vi "TechnosoftVariables.vi"(0 "error in (no error)":errorcluster) -> (1 "error out":errorcluster, 3 "Decoded new":bool, 4 "TSM variable table":T1 {"?" format="%x"})   [LabVIEW 8.6]
panel:
  out "Number of variables":i32
  out "Numeric":i32
  out "decode":string
  out "Unknown type String":string
  in  "Firmware variables.cfg":string
  # "Store as a constant!\nMap data 0000-FFFF\nEPROM: 10000-1FFFF\nTSM prog: 20000-2FFFF"
  # "TSM Data: 200-3FF and 800-9FF-FFF, 8000-FFFF(external)\nTSM prog: 8000-FFFF\nEPROM:  4000-7FFF"
  # "In the Technosoft manual all real variables are CAPITAL letters,\nso do it here."
  # "checked with old dataset: i2tintlim_m and other _m"
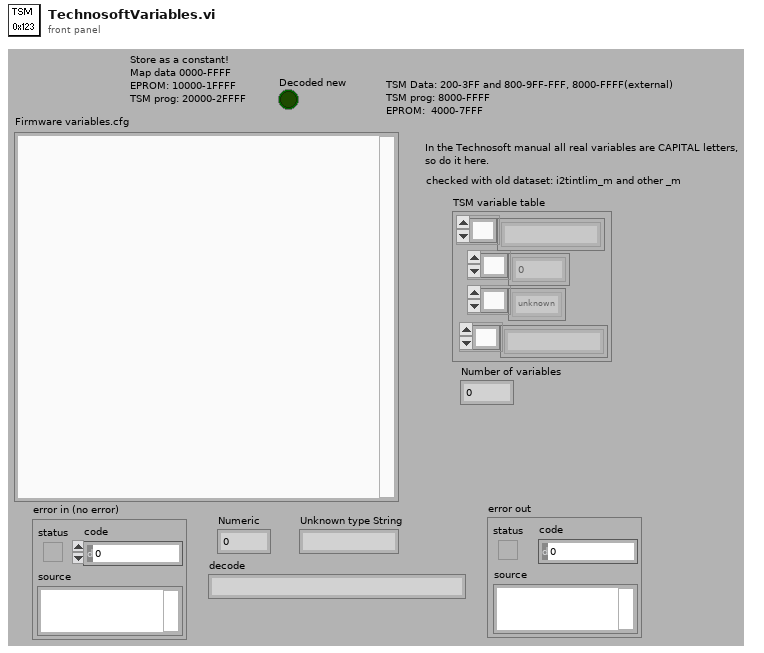
[diagram p1: front panel]
types:
  T1 = cluster{string[], u32[], enum16{"unknown", "i16", "u16", "i32", "u32", "fix32"}[], "comment":string[]}
  T2 = cluster{"String 1":string, i32, "type":enum16{"unknown", "i16", "u16", "i32", "u32", "fix32"}, "trimmed string":string}[]
  T3 = enum16{"unknown", "i16", "u16", "i32", "u32", "fix32"}[]
  T4 = enum16{"unknown", "i16", "u16", "i32", "u32", "fix32"}
  T5 = cluster{string, "Address":u32, "type":enum16{"unknown", "i16", "u16", "i32", "u32", "fix32"}, "trimmed string":string}
  T6 = cluster{"String 1":string, "Address":u32, "type":enum16{"unknown", "i16", "u16", "i32", "u32", "fix32"}, "trimmed string":string}[]
  T7 = cluster{string[], u32[], enum16{"unknown", "i16", "u16", "i32", "u32", "fix32"}[], string[]}
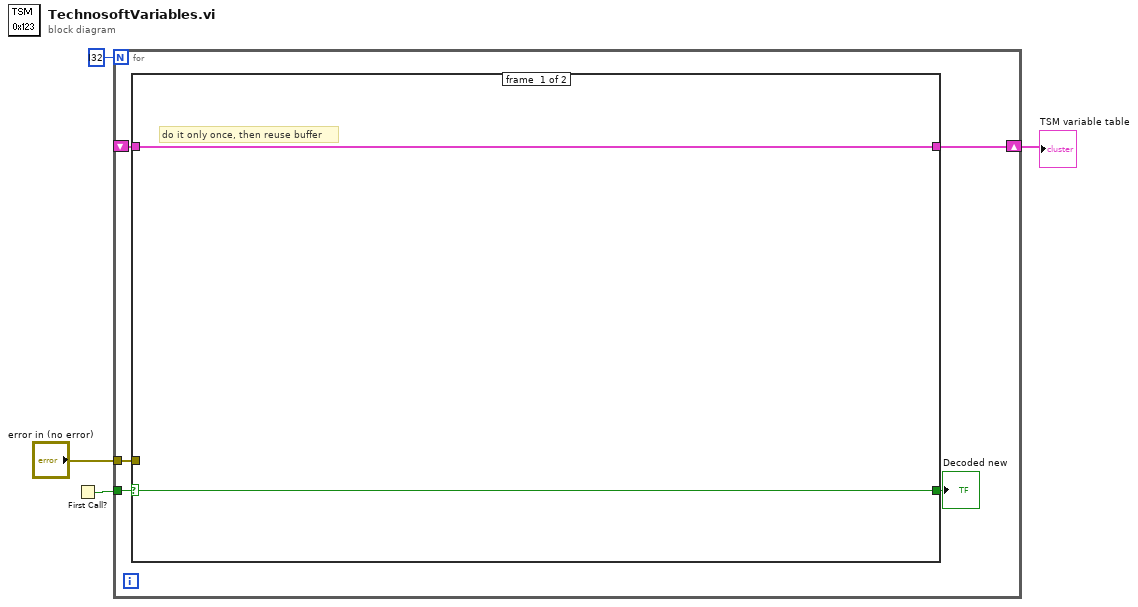
[diagram p0: block diagram]
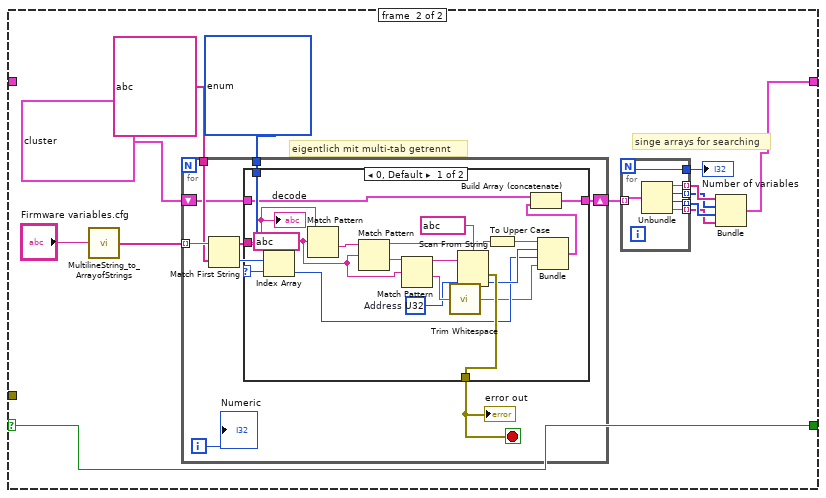
[diagram p2: hidden frame]
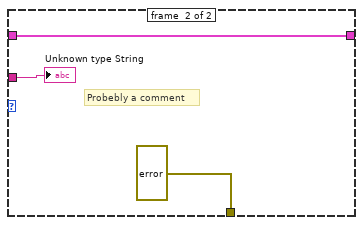
[diagram p3: hidden frame]
diagram:
  n1 = First Call?() -> (First Call?: T/F=w4:bool)
  n2 = for {
    N: i32 ? -> [_]
    tunnel: w4 -> [w9]
    tunnel: "error in (no error)" -> [w7]
    shift-right: [w6] -> w2
    shift-left: _ -> [w5]
    n3 = case shown="True" w9 {
      selector: w9 -> [w11 w20]
      tunnel: [w11 w20] -> w8
      tunnel: w7 -> [_ _]
      tunnel: [w10 w13] -> w6
      tunnel: w5 -> [w10 _]
      frame #0 {
        # "do it only once, then reuse buffer"
      }
      frame #1 {
        w21 = T3 ? items=["unknown", "i16", "u16", "i32", "u32", "fix32"]
        # "singe arrays for searching"
        # "eigentlich mit multi-tab getrennt"
        n4 = call "MultilineString_to_ArrayofStrings.vi"("String 1"="Firmware variables.cfg") -> ("String Array"=w23:string[])  [unwired: 1 in]
        n5 = for {
          tunnel: w23 -> [w39] mode=indexing
          tunnel: string[] ? -> [w38]
          tunnel: w21 -> [w35]
          shift-right: [w32] -> w18
          shift-left: T2 ? -> [w31]
          i -> [w33]
          stop <- w34 stop-if-true
          n6 = Match First String(2:w38, 3:w39) -> (0:w37:i32, 1:w36:string)
          n7 = case shown="0, Default" w37 {
            selector: w37 -> [w57 _]
            tunnel: w36 -> [w56 w61]
            tunnel: w35 -> [w58 _]
            tunnel: [w49 errorcluster ? ("error IO")] -> w34
            tunnel: [w46 w59] -> w32
            tunnel: w31 -> [w43 w59]
            frame #0 {
              w42 = u32 ?  # Address
              w53 = string ? ("regular expression")
              n8 = Index Array(array=w58, index=w57) -> (element=w45:T4)
              n9 = Match Pattern(string=w56, regular expression=w53) -> (after substring=w55:string)  [unwired: 4 out]
              n10 = Match Pattern(string=w55, regular expression=w53) -> (before substring=w41:string, after substring=w54:string)  [unwired: 3 out]
              n11 = Match Pattern(string=w54, regular expression=w53) -> (before substring=w51:string, after substring=w52:string)  [unwired: 3 out]
              n12 = call <vilib>:"Trim Whitespace.vi"("string"=w52) -> ("trimmed string"=w44:string)  [unwired: 1 in]
              n13 = Scan From String(format string=string ?, input string=w51, default 1=w42) -> (error out=w49:errorcluster, output 1=w48:u32)  [unwired: 2 in, 2 out]
              n14 = To Upper Case(1:w41) -> (0:w40:string)
              n15 = Bundle(w40, "Address"=w48, "type"=w45, "trimmed string"=w44) -> (w47:T5)  [unwired: 1 out]
              n16 = Build Array (concatenate)(w43, w47) -> (w46:T6)
              "decode" <- w56
            }
            frame #1 {
              # "Probebly a comment"
              "Unknown type String" <- w61
            }
          }
          "error out" <- w34
          "Numeric" <- w33
        }
        n17 = for {
          N -> [w25]
          tunnel: w18 -> [w30] mode=indexing
          tunnel: [w29] -> w17 mode=indexing
          tunnel: [w28] -> w16 mode=indexing
          tunnel: [w27] -> w15 mode=indexing
          tunnel: [w26] -> w12 mode=indexing
          tunnel: [w25] -> w14
          n18 = Unbundle(w30) -> ("String 1"=w29:string, "Address"=w28:u32, "type"=w27:T4, "trimmed string"=w26:string)
        }
        "Number of variables" <- w14
        n19 = Bundle(w17, w16, w15, w12) -> (w13:T7)  [unwired: 1 out]
      }
    }
    "Decoded new" <- w8
  }
  "TSM variable table" <- w2
